vi "I-V扫描脚本.vi"(1 "参数":T1) -> (0 "Script":string)   [LabVIEW 2020]
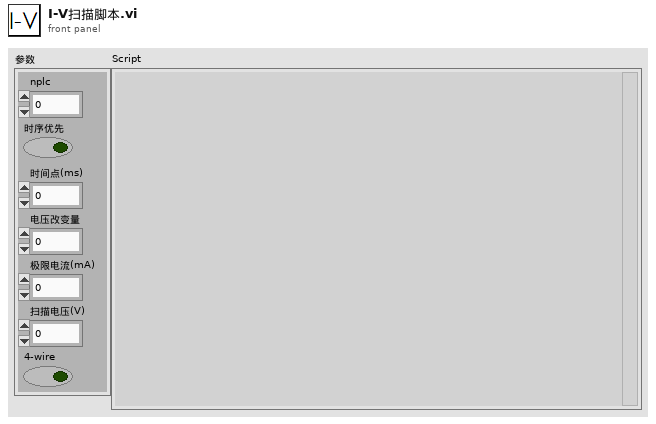
[diagram p1: front panel]
types:
  T1 = cluster{"nplc":dbl, "时序优先":bool, "时间点(ms)":dbl, "电压改变量":dbl, "极限电流(mA)":dbl, "扫描电压(V)":dbl, "4-wire":bool}
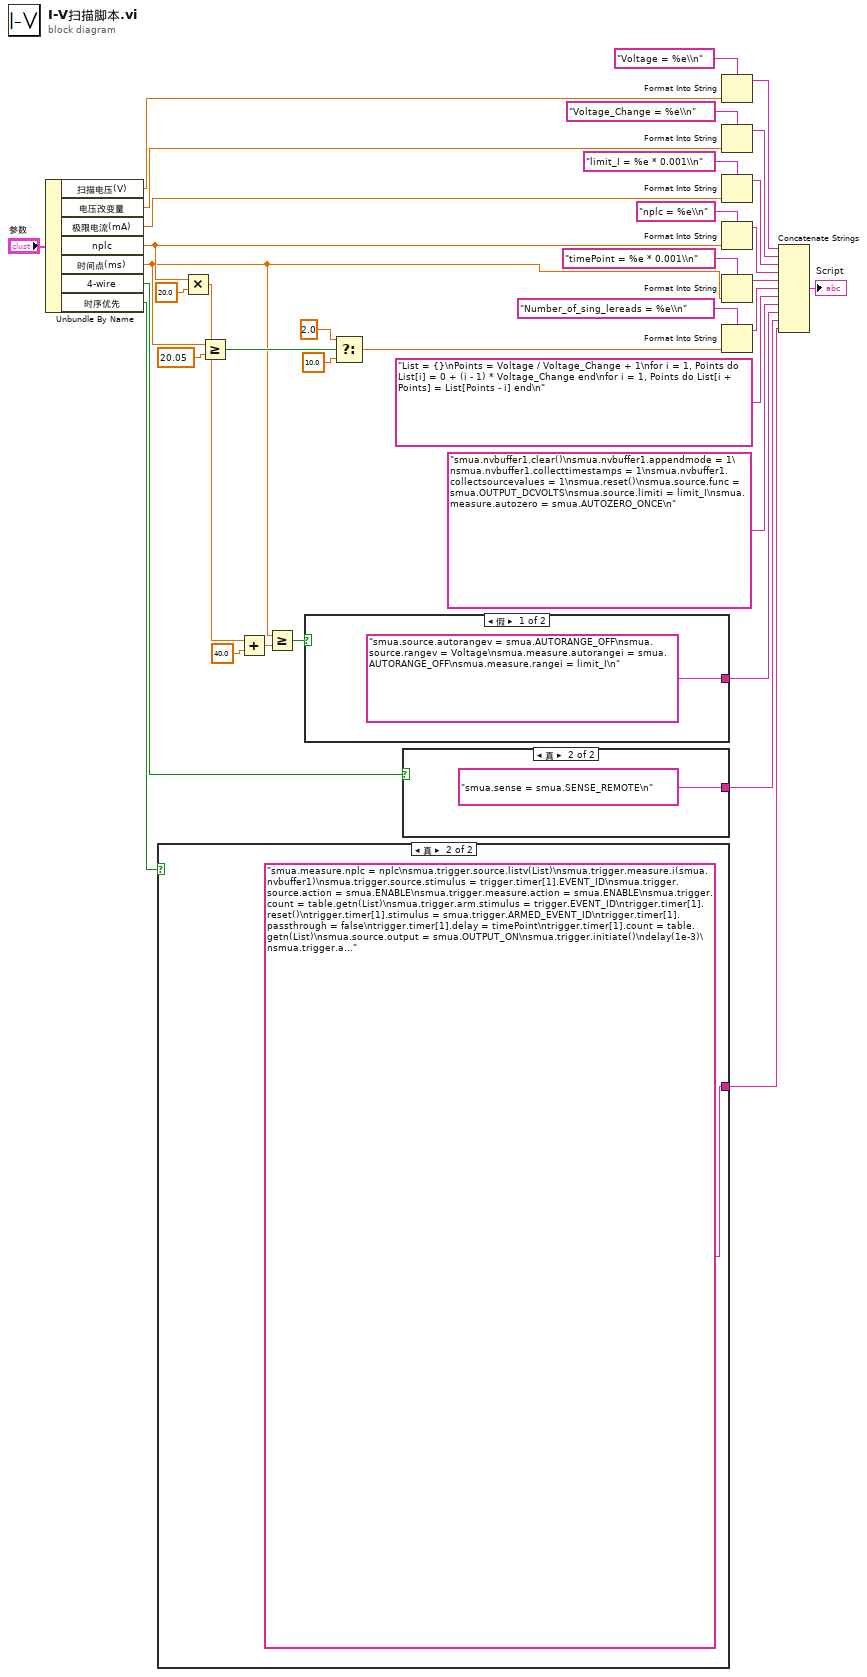
[diagram p0: block diagram]
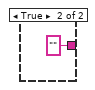
[diagram p2: hidden frame]
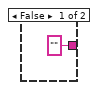
[diagram p3: hidden frame]
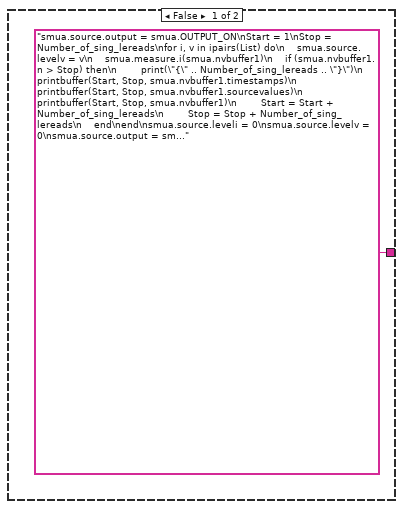
[diagram p4: hidden frame]
diagram:
  n1 = Unbundle By Name("参数") -> ("扫描电压(V)"=w23:dbl, "电压改变量"=w22:dbl, "极限电流(mA)"=w21:dbl, "nplc"=w5:dbl, "时间点(ms)"=w1:dbl, "4-wire"=w20:bool, "时序优先"=w19:bool)
  n2 = case shown="真" w19 {
    tunnel: ["smua.source.output = smua.OUTPUT_ON\nStart = 1\nStop = Number_of_sing_lereads\nfor i, v in ipairs(List) do\n    smua.source.levelv = v\n    smua.measure.i(smua.nvbuffer1)\n    if (smua.nvbuffer1.n > Stop) then\n        print(\"{\" .. Number_of_sing_lereads .. \"}\")\n        printbuffer(Start, Stop, smua.nvbuffer1.timestamps)\n        printbuffer(Start, Stop, smua.nvbuffer1.sourcevalues)\n        printbuffer(Start, Stop, smua.nvbuffer1)\n        Start = Start + Number_of_sing_lereads\n        Stop = Stop + Number_of_sing_lereads\n    end\nend\nsmua.source.leveli = 0\nsmua.source.levelv = 0\nsmua.source.output = smua.OUTPUT_OFF\nStop = table.getn(List)\nprint(\"{\" .. Stop - Start + 1 .. \"}\")\nprintbuffer(Start, Stop, smua.nvbuffer1.timestamps)\nprintbuffer(Start, Stop, smua.nvbuffer1.sourcevalues)\nprintbuffer(Start, Stop, smua.nvbuffer1)\nprint(\"{done}\")\nreset()\n" "smua.measure.nplc = nplc\nsmua.trigger.source.listv(List)\nsmua.trigger.measure.i(smua.nvbuffer1)\nsmua.trigger.source.stimulus = trigger.timer[1].EVENT_ID\nsmua.trigger.source.action = smua.ENABLE\nsmua.trigger.measure.action = smua.ENABLE\nsmua.trigger.count = table.getn(List)\nsmua.trigger.arm.stimulus = trigger.EVENT_ID\ntrigger.timer[1].reset()\ntrigger.timer[1].stimulus = smua.trigger.ARMED_EVENT_ID\ntrigger.timer[1].passthrough = false\ntrigger.timer[1].delay = timePoint\ntrigger.timer[1].count = table.getn(List)\nsmua.source.output = smua.OUTPUT_ON\nsmua.trigger.initiate()\ndelay(1e-3)\nsmua.trigger.arm.set()\nfunction _done()\n    Start = 1\n    Stop = Number_of_sing_lereads\n    repeat\n        if (bit.test(status.operation.instrument.smua.condition, 4) == false) then\n            smua.source.leveli = 0\n            smua.source.levelv = 0\n            smua.source.output = smua.OUTPUT_OFF\n            Stop = table.getn(List)\n            print(\"{\" .. Stop - Start + 1 .. \"}\")\n            printbuffer(Start, Stop, smua.nvbuffer1.timestamps)\n            printbuffer(Start, Stop, smua.nvbuffer1.sourcevalues)\n            printbuffer(Start, Stop, smua.nvbuffer1)\n            print(\"{done}\")\n            return\n        elseif (smua.nvbuffer1.n > Stop) then\n            print(\"{\" .. Number_of_sing_lereads .. \"}\")\n            printbuffer(Start, Stop, smua.nvbuffer1.timestamps)\n            printbuffer(Start, Stop, smua.nvbuffer1.sourcevalues)\n            printbuffer(Start, Stop, smua.nvbuffer1)\n            Start = Start + Number_of_sing_lereads\n            Stop = Stop + Number_of_sing_lereads\n        end\n        delay(timePoint)\n    until (false)\nend\n_done()\nreset()\n"] -> w18
    frame False {
    }
    frame True {
    }
  }
  n3 = Multiply(x=w5, y=20.0) -> (x*y=w8:dbl)
  n4 = Greater Or Equal?(x=w1, y=20.05) -> (x >= y?=w13:bool)
  n5 = Add(x=w8, y=40.0) -> (x+y=w6:dbl)
  n6 = Greater Or Equal?(x=w1, y=w6) -> (x >= y?=w4:bool)
  n7 = case shown="假" w4 {
    tunnel: ["smua.source.autorangev = smua.AUTORANGE_OFF\nsmua.source.rangev = Voltage\nsmua.measure.autorangei = smua.AUTORANGE_OFF\nsmua.measure.rangei = limit_I\n" ""] -> w3
    frame False {
    }
    frame True {
    }
  }
  n8 = Select(t=2.0, s=w13, f=10.0) -> (s? t:f=w10:dbl)
  n9 = case shown="真" w20 {
    tunnel: ["" "smua.sense = smua.SENSE_REMOTE\n"] -> w2
    frame False {
    }
    frame True {
    }
  }
  n10 = Format Into String(format string="Voltage = %e\\n" ("格式字符串"), w23) -> (resulting string=w33:string)  [unwired: 2 in, 1 out]
  n11 = Format Into String(format string="Voltage_Change = %e\\n" ("格式字符串"), w22) -> (resulting string=w31:string)  [unwired: 2 in, 1 out]
  n12 = Format Into String(format string="limit_I = %e * 0.001\\n" ("格式字符串"), w21) -> (resulting string=w30:string)  [unwired: 2 in, 1 out]
  n13 = Format Into String(format string="nplc = %e\\n", w5) -> (resulting string=w28:string)  [unwired: 2 in, 1 out]
  n14 = Format Into String(format string="timePoint = %e * 0.001\\n", w1) -> (resulting string=w26:string)  [unwired: 2 in, 1 out]
  n15 = Format Into String(format string="Number_of_sing_lereads = %e\\n" ("格式字符串"), w10) -> (resulting string=w16:string)  [unwired: 2 in, 1 out]
  n16 = Concatenate Strings(w33, w31, w30, w28, w26, w16, "List = {}\nPoints = Voltage / Voltage_Change + 1\nfor i = 1, Points do List[i] = 0 + (i - 1) * Voltage_Change end\nfor i = 1, Points do List[i + Points] = List[Points - i] end\n", "smua.nvbuffer1.clear()\nsmua.nvbuffer1.appendmode = 1\nsmua.nvbuffer1.collecttimestamps = 1\nsmua.nvbuffer1.collectsourcevalues = 1\nsmua.reset()\nsmua.source.func = smua.OUTPUT_DCVOLTS\nsmua.source.limiti = limit_I\nsmua.measure.autozero = smua.AUTOZERO_ONCE\n", w3, w2, w18) -> (→"Script":string)
